vi "Get Localhost Name.vi"(8 "error in (no error)":errorcluster, 11 "Parent in":refnum<class "Message_Distributor_Class.lvclass">) -> (0 "error out":errorcluster, 1 "PC Name":string, 3 "Parent out":refnum<class "Message_Distributor_Class.lvclass">)   [LabVIEW 2023, in "Actor_Message_Distributor.lvlib" / "Message_Distributor_Class.lvclass"]
uses:
  Message_Distributor_Class.lvclass
  Abstraction_Interface_Class/Abstraction_Interface_Class.lvclass
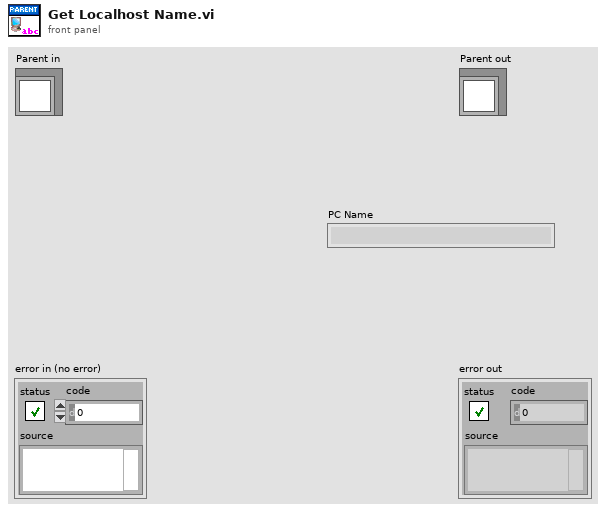
[diagram p1: front panel]
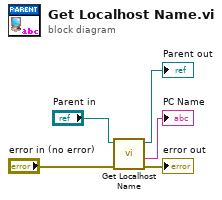
[diagram p0: block diagram]
diagram:
  n1 = call-parent "Get Localhost Name.vi"("error in (no error)"="error in (no error)", "Interface_Class in"="Parent in") -> ("error out"=→"error out":errorcluster, "PC Name"=→"PC Name":string, "Interface_Class out"=→"Parent out":refnum<class "Message_Distributor_Class.lvclass">)  [unwired: 7 in]
